vi "Operate.vi"(0 "Multiply in":refnum<class "Multiply.lvclass">, 11 "error in (no error)":errorcluster) -> (4 "Multiply out":refnum<class "Multiply.lvclass">, 15 "error out":errorcluster)   [LabVIEW 2020, in "Multiply.lvclass"]
uses:
  Multiply.lvclass
  C:/Users/khishore.kumar/Khishore/labview_tips_2024/src/Assignment 25/Arithmetic Operations/Arithmetic Operations.lvclass
  Arithmetic Operations.lvclass/Arithmetic Operations.ctl
  Accessors/Read/Read A.vi
  Accessors/Read/Read B.vi
  Accessors/Write/Write C.vi
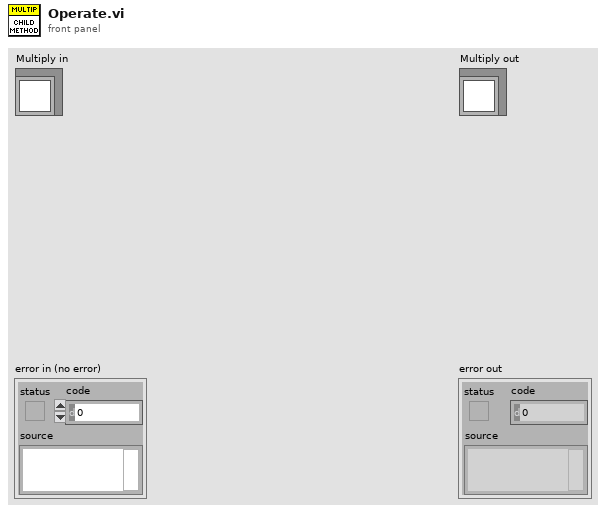
[diagram p1: front panel]
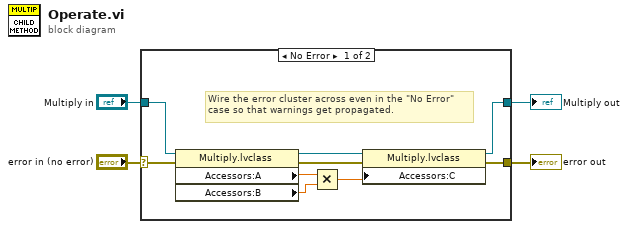
[diagram p0: block diagram]
diagram:
  n1 = case shown="No Error" "error in (no error)" {
    selector: "error in (no error)" -> [w13 w15]
    tunnel: [w11 w15] -> w3
    tunnel: [w8 w14] -> w1
    tunnel: "Multiply in" -> [w10 w14]
    frame No Error {
      # "Wire the error cluster across even in the \"No Error\"\ncase so that warnings get propagated."
      n2 = property class="Multiply.lvclass"(reference=w10, error in=w13) -> (reference out=w9:refnum<class "Multiply.lvclass">, error out=w12:errorcluster, "Accessors:A"=w5:dbl, "Accessors:B"=w6:dbl)
      n3 = Multiply(x=w5, y=w6) -> (x*y=w7:dbl)
      n4 = property class="Multiply.lvclass"(reference=w9, error in=w12, "Accessors:C"=w7) -> (reference out=w8:refnum<class "Multiply.lvclass">, error out=w11:errorcluster)
    }
    frame Error {
    }
  }
  "error out" <- w3
  "Multiply out" <- w1
